vi "PXI Pnuematic Control.vi"(1 "Enable Relays":bool, 2 "Reset IO":bool, 3 "error in (no error)":errorcluster {"code" format="%.0x"}, 4 "Enum":T2(ring), 5 "topology name":T1="2566/16-SPDT", 6 "resource name":refnum<k15>="PXI1Slot6") -> (0 "error out":errorcluster)   [LabVIEW 2014]
uses:
  <instrlib>/niSwitch/niswitch.llb/niSwitch Relay Action.ctl
  <instrlib>/niSwitch/niswitch.llb/niSwitch Topologies.ctl
panel:
  out "instrument handle out":refnum<k15>
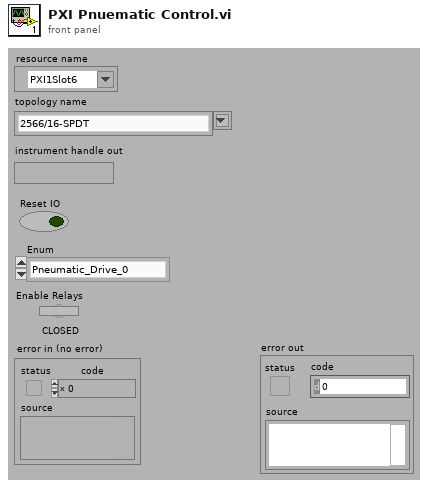
[diagram p1: front panel]
types:
  T1 = typedef "niSwitch Topologies.ctl" = string
  T2 = enum16{"Pneumatic_Drive_0", "Pneumatic_Drive_1", "Pneumatic_Drive_2", "Pneumatic_Drive_3", "Pneumatic_Drive_4", "Pneumatic_Drive_5", "Pneumatic_Drive_6", "Pneumatic_Drive_7", "Pneumatic_Drive_8", "Pneumatic_Drive_9", "Pneumatic_Drive_10", "Pneumatic_Drive_11", "Pneumatic_Drive_12", "Pneumatic_Drive_13", "Pneumatic_Drive_14", "Pneumatic_Drive_15", "Init Pneumatic Relays", "DeInit Pneumatic Relays"}
  T3 = typedef "niSwitch Relay Action.ctl" = i32
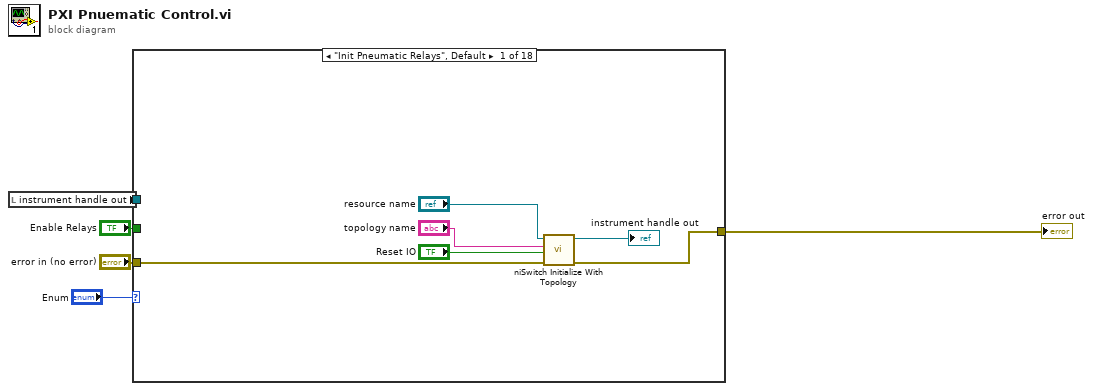
[diagram p0: block diagram]
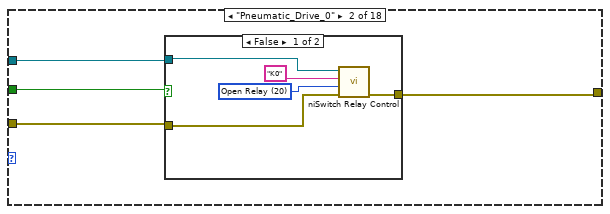
[diagram p2: hidden frame]
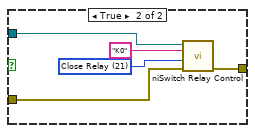
[diagram p3: hidden frame]
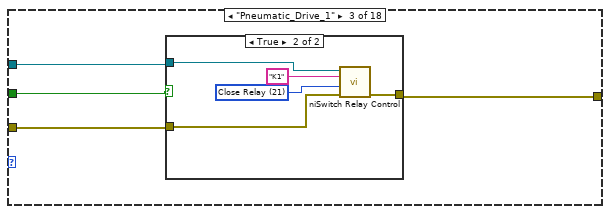
[diagram p4: hidden frame]
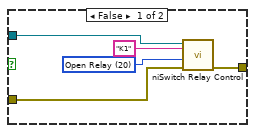
[diagram p5: hidden frame]
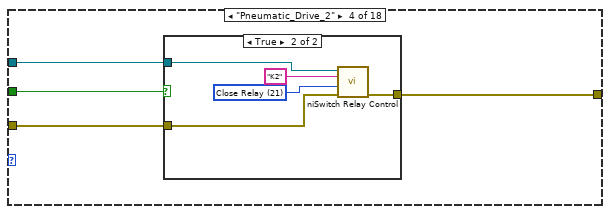
[diagram p6: hidden frame]
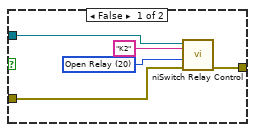
[diagram p7: hidden frame]
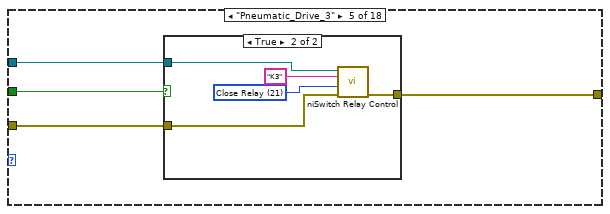
[diagram p8: hidden frame]
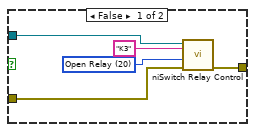
[diagram p9: hidden frame]
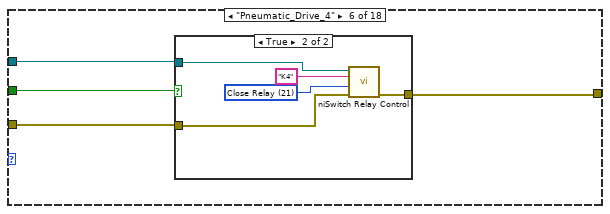
[diagram p10: hidden frame]
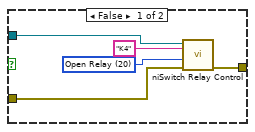
[diagram p11: hidden frame]
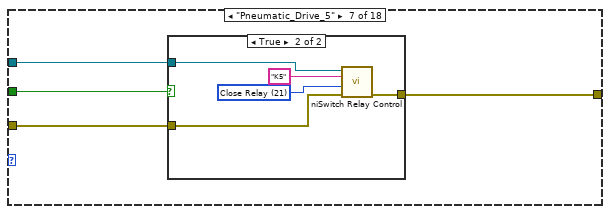
[diagram p12: hidden frame]
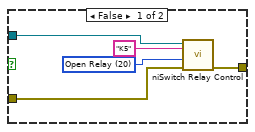
[diagram p13: hidden frame]
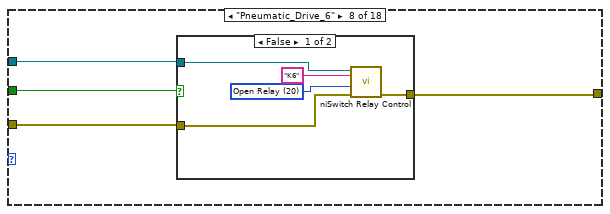
[diagram p14: hidden frame]
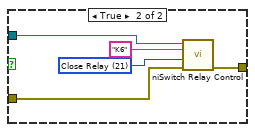
[diagram p15: hidden frame]
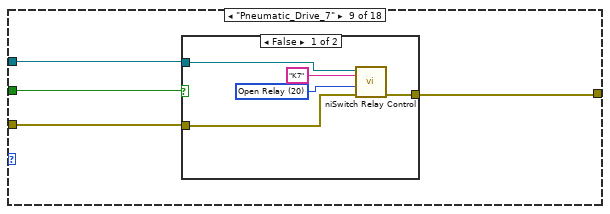
[diagram p16: hidden frame]
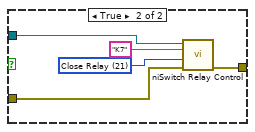
[diagram p17: hidden frame]
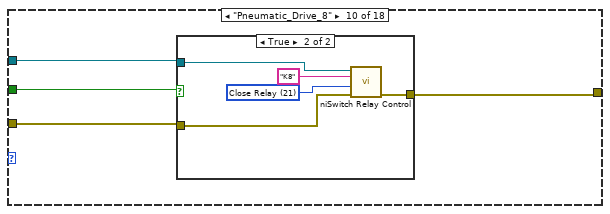
[diagram p18: hidden frame]
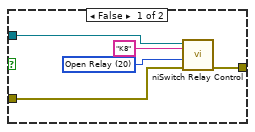
[diagram p19: hidden frame]
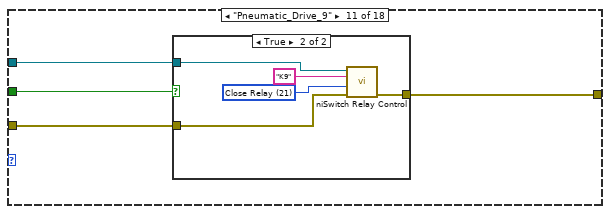
[diagram p20: hidden frame]
diagram:
  n1 = local read "instrument handle out"() -> (w4:refnum<k15>)
  n2 = case shown="\"Init Pneumatic Relays\", Default" "Enum" {
    tunnel: w4 -> [_ w15 w29 w43 w57 w71 w85 w99 w113 w127 w141 w155 w169 w183 w197 w211 w225 w238]
    tunnel: [w11 w12 w26 w40 w54 w68 w82 w96 w110 w124 w138 w152 w166 w180 w194 w208 w222 w236] -> w3
    tunnel: "Enable Relays" -> [_ w14 w27 w42 w56 w70 w84 w98 w112 w126 w140 w154 w168 w182 w196 w210 w224 _]
    tunnel: "error in (no error)" -> [w10 w13 w28 w41 w55 w69 w83 w97 w111 w125 w139 w153 w167 w181 w195 w209 w223 w237]
    frame "Init Pneumatic Relays", Default {
      n3 = call <instrlib>:"niSwitch Initialize With Topology.vi"("error in (no error)"=w10, "reset device (boolean value)"="Reset IO", "topology name"="topology name", "resource name"="resource name") -> ("error out"=w11:errorcluster, "instrument handle out"=→"instrument handle out":refnum<k15>)  [unwired: 6 in]
    }
    frame "Pneumatic_Drive_0" {
      n4 = case shown="False" w14 {
        tunnel: w15 -> [w18 w22]
        tunnel: [w19 w23] -> w12
        tunnel: w13 -> [w17 w21]
        frame False {
          w20 = T3 20 items=["Open Relay"=20, "Close Relay"=21] ("relay action (Close Relay)")
          n5 = call <instrlib>:"niSwitch Relay Control.vi"("error in (no error)"=w17, "relay action (Close Relay)"=w20, "relay name"="K0", "instrument handle"=w18) -> ("error out"=w19:errorcluster)  [unwired: 6 in, 1 out]
        }
        frame True {
          w25 = T3 21 items=["Open Relay"=20, "Close Relay"=21] ("relay action (Close Relay)")
          n6 = call <instrlib>:"niSwitch Relay Control.vi"("error in (no error)"=w21, "relay action (Close Relay)"=w25, "relay name"="K0", "instrument handle"=w22) -> ("error out"=w23:errorcluster)  [unwired: 6 in, 1 out]
        }
      }
    }
    frame "Pneumatic_Drive_1" {
      n7 = case shown="True" w27 {
        tunnel: w29 -> [w31 w36]
        tunnel: [w32 w37] -> w26
        tunnel: w28 -> [w30 w35]
        frame False {
          w34 = T3 20 items=["Open Relay"=20, "Close Relay"=21] ("relay action (Close Relay)")
          n8 = call <instrlib>:"niSwitch Relay Control.vi"("error in (no error)"=w30, "relay action (Close Relay)"=w34, "relay name"="K1", "instrument handle"=w31) -> ("error out"=w32:errorcluster)  [unwired: 6 in, 1 out]
        }
        frame True {
          w39 = T3 21 items=["Open Relay"=20, "Close Relay"=21] ("relay action (Close Relay)")
          n9 = call <instrlib>:"niSwitch Relay Control.vi"("error in (no error)"=w35, "relay action (Close Relay)"=w39, "relay name"="K1", "instrument handle"=w36) -> ("error out"=w37:errorcluster)  [unwired: 6 in, 1 out]
        }
      }
    }
    frame "Pneumatic_Drive_2" {
      n10 = case shown="True" w42 {
        tunnel: w43 -> [w45 w50]
        tunnel: [w46 w51] -> w40
        tunnel: w41 -> [w44 w49]
        frame False {
          w48 = T3 20 items=["Open Relay"=20, "Close Relay"=21] ("relay action (Close Relay)")
          n11 = call <instrlib>:"niSwitch Relay Control.vi"("error in (no error)"=w44, "relay action (Close Relay)"=w48, "relay name"="K2", "instrument handle"=w45) -> ("error out"=w46:errorcluster)  [unwired: 6 in, 1 out]
        }
        frame True {
          w53 = T3 21 items=["Open Relay"=20, "Close Relay"=21] ("relay action (Close Relay)")
          n12 = call <instrlib>:"niSwitch Relay Control.vi"("error in (no error)"=w49, "relay action (Close Relay)"=w53, "relay name"="K2", "instrument handle"=w50) -> ("error out"=w51:errorcluster)  [unwired: 6 in, 1 out]
        }
      }
    }
    frame "Pneumatic_Drive_3" {
      n13 = case shown="True" w56 {
        tunnel: w57 -> [w59 w64]
        tunnel: [w60 w65] -> w54
        tunnel: w55 -> [w58 w63]
        frame False {
          w62 = T3 20 items=["Open Relay"=20, "Close Relay"=21] ("relay action (Close Relay)")
          n14 = call <instrlib>:"niSwitch Relay Control.vi"("error in (no error)"=w58, "relay action (Close Relay)"=w62, "relay name"="K3", "instrument handle"=w59) -> ("error out"=w60:errorcluster)  [unwired: 6 in, 1 out]
        }
        frame True {
          w67 = T3 21 items=["Open Relay"=20, "Close Relay"=21] ("relay action (Close Relay)")
          n15 = call <instrlib>:"niSwitch Relay Control.vi"("error in (no error)"=w63, "relay action (Close Relay)"=w67, "relay name"="K3", "instrument handle"=w64) -> ("error out"=w65:errorcluster)  [unwired: 6 in, 1 out]
        }
      }
    }
    frame "Pneumatic_Drive_4" {
      n16 = case shown="True" w70 {
        tunnel: w71 -> [w73 w78]
        tunnel: [w74 w79] -> w68
        tunnel: w69 -> [w72 w77]
        frame False {
          w76 = T3 20 items=["Open Relay"=20, "Close Relay"=21] ("relay action (Close Relay)")
          n17 = call <instrlib>:"niSwitch Relay Control.vi"("error in (no error)"=w72, "relay action (Close Relay)"=w76, "relay name"="K4", "instrument handle"=w73) -> ("error out"=w74:errorcluster)  [unwired: 6 in, 1 out]
        }
        frame True {
          w81 = T3 21 items=["Open Relay"=20, "Close Relay"=21] ("relay action (Close Relay)")
          n18 = call <instrlib>:"niSwitch Relay Control.vi"("error in (no error)"=w77, "relay action (Close Relay)"=w81, "relay name"="K4", "instrument handle"=w78) -> ("error out"=w79:errorcluster)  [unwired: 6 in, 1 out]
        }
      }
    }
    frame "Pneumatic_Drive_5" {
      n19 = case shown="True" w84 {
        tunnel: w85 -> [w87 w92]
        tunnel: [w88 w93] -> w82
        tunnel: w83 -> [w86 w91]
        frame False {
          w90 = T3 20 items=["Open Relay"=20, "Close Relay"=21] ("relay action (Close Relay)")
          n20 = call <instrlib>:"niSwitch Relay Control.vi"("error in (no error)"=w86, "relay action (Close Relay)"=w90, "relay name"="K5", "instrument handle"=w87) -> ("error out"=w88:errorcluster)  [unwired: 6 in, 1 out]
        }
        frame True {
          w95 = T3 21 items=["Open Relay"=20, "Close Relay"=21] ("relay action (Close Relay)")
          n21 = call <instrlib>:"niSwitch Relay Control.vi"("error in (no error)"=w91, "relay action (Close Relay)"=w95, "relay name"="K5", "instrument handle"=w92) -> ("error out"=w93:errorcluster)  [unwired: 6 in, 1 out]
        }
      }
    }
    frame "Pneumatic_Drive_6" {
      n22 = case shown="False" w98 {
        tunnel: w99 -> [w101 w106]
        tunnel: [w102 w107] -> w96
        tunnel: w97 -> [w100 w105]
        frame False {
          w104 = T3 20 items=["Open Relay"=20, "Close Relay"=21] ("relay action (Close Relay)")
          n23 = call <instrlib>:"niSwitch Relay Control.vi"("error in (no error)"=w100, "relay action (Close Relay)"=w104, "relay name"="K6", "instrument handle"=w101) -> ("error out"=w102:errorcluster)  [unwired: 6 in, 1 out]
        }
        frame True {
          w109 = T3 21 items=["Open Relay"=20, "Close Relay"=21] ("relay action (Close Relay)")
          n24 = call <instrlib>:"niSwitch Relay Control.vi"("error in (no error)"=w105, "relay action (Close Relay)"=w109, "relay name"="K6", "instrument handle"=w106) -> ("error out"=w107:errorcluster)  [unwired: 6 in, 1 out]
        }
      }
    }
    frame "Pneumatic_Drive_7" {
      n25 = case shown="False" w112 {
        tunnel: w113 -> [w115 w120]
        tunnel: [w116 w121] -> w110
        tunnel: w111 -> [w114 w119]
        frame False {
          w118 = T3 20 items=["Open Relay"=20, "Close Relay"=21] ("relay action (Close Relay)")
          n26 = call <instrlib>:"niSwitch Relay Control.vi"("error in (no error)"=w114, "relay action (Close Relay)"=w118, "relay name"="K7", "instrument handle"=w115) -> ("error out"=w116:errorcluster)  [unwired: 6 in, 1 out]
        }
        frame True {
          w123 = T3 21 items=["Open Relay"=20, "Close Relay"=21] ("relay action (Close Relay)")
          n27 = call <instrlib>:"niSwitch Relay Control.vi"("error in (no error)"=w119, "relay action (Close Relay)"=w123, "relay name"="K7", "instrument handle"=w120) -> ("error out"=w121:errorcluster)  [unwired: 6 in, 1 out]
        }
      }
    }
    frame "Pneumatic_Drive_8" {
      n28 = case shown="True" w126 {
        tunnel: w127 -> [w129 w134]
        tunnel: [w130 w135] -> w124
        tunnel: w125 -> [w128 w133]
        frame False {
          w132 = T3 20 items=["Open Relay"=20, "Close Relay"=21] ("relay action (Close Relay)")
          n29 = call <instrlib>:"niSwitch Relay Control.vi"("error in (no error)"=w128, "relay action (Close Relay)"=w132, "relay name"="K8", "instrument handle"=w129) -> ("error out"=w130:errorcluster)  [unwired: 6 in, 1 out]
        }
        frame True {
          w137 = T3 21 items=["Open Relay"=20, "Close Relay"=21] ("relay action (Close Relay)")
          n30 = call <instrlib>:"niSwitch Relay Control.vi"("error in (no error)"=w133, "relay action (Close Relay)"=w137, "relay name"="K8", "instrument handle"=w134) -> ("error out"=w135:errorcluster)  [unwired: 6 in, 1 out]
        }
      }
    }
    frame "Pneumatic_Drive_9" {
      n31 = case shown="True" w140 {
        tunnel: w141 -> [w143 w148]
        tunnel: [w144 w149] -> w138
        tunnel: w139 -> [w142 w147]
        frame False {
          w146 = T3 20 items=["Open Relay"=20, "Close Relay"=21] ("relay action (Close Relay)")
          n32 = call <instrlib>:"niSwitch Relay Control.vi"("error in (no error)"=w142, "relay action (Close Relay)"=w146, "relay name"="K9", "instrument handle"=w143) -> ("error out"=w144:errorcluster)  [unwired: 6 in, 1 out]
        }
        frame True {
          w151 = T3 21 items=["Open Relay"=20, "Close Relay"=21] ("relay action (Close Relay)")
          n33 = call <instrlib>:"niSwitch Relay Control.vi"("error in (no error)"=w147, "relay action (Close Relay)"=w151, "relay name"="K9", "instrument handle"=w148) -> ("error out"=w149:errorcluster)  [unwired: 6 in, 1 out]
        }
      }
    }
    frame "Pneumatic_Drive_10" {
      n34 = case shown="True" w154 {
        tunnel: w155 -> [w157 w162]
        tunnel: [w158 w163] -> w152
        tunnel: w153 -> [w156 w161]
        frame False {
          w160 = T3 20 items=["Open Relay"=20, "Close Relay"=21] ("relay action (Close Relay)")
          n35 = call <instrlib>:"niSwitch Relay Control.vi"("error in (no error)"=w156, "relay action (Close Relay)"=w160, "relay name"="K10", "instrument handle"=w157) -> ("error out"=w158:errorcluster)  [unwired: 6 in, 1 out]
        }
        frame True {
          w165 = T3 21 items=["Open Relay"=20, "Close Relay"=21] ("relay action (Close Relay)")
          n36 = call <instrlib>:"niSwitch Relay Control.vi"("error in (no error)"=w161, "relay action (Close Relay)"=w165, "relay name"="K10", "instrument handle"=w162) -> ("error out"=w163:errorcluster)  [unwired: 6 in, 1 out]
        }
      }
    }
    frame "Pneumatic_Drive_11" {
      n37 = case shown="True" w168 {
        tunnel: w169 -> [w171 w176]
        tunnel: [w172 w177] -> w166
        tunnel: w167 -> [w170 w175]
        frame False {
          w174 = T3 20 items=["Open Relay"=20, "Close Relay"=21] ("relay action (Close Relay)")
          n38 = call <instrlib>:"niSwitch Relay Control.vi"("error in (no error)"=w170, "relay action (Close Relay)"=w174, "relay name"="K11", "instrument handle"=w171) -> ("error out"=w172:errorcluster)  [unwired: 6 in, 1 out]
        }
        frame True {
          w179 = T3 21 items=["Open Relay"=20, "Close Relay"=21] ("relay action (Close Relay)")
          n39 = call <instrlib>:"niSwitch Relay Control.vi"("error in (no error)"=w175, "relay action (Close Relay)"=w179, "relay name"="K11", "instrument handle"=w176) -> ("error out"=w177:errorcluster)  [unwired: 6 in, 1 out]
        }
      }
    }
    frame "Pneumatic_Drive_12" {
      n40 = case shown="True" w182 {
        tunnel: w183 -> [w185 w190]
        tunnel: [w186 w191] -> w180
        tunnel: w181 -> [w184 w189]
        frame False {
          w188 = T3 20 items=["Open Relay"=20, "Close Relay"=21] ("relay action (Close Relay)")
          n41 = call <instrlib>:"niSwitch Relay Control.vi"("error in (no error)"=w184, "relay action (Close Relay)"=w188, "relay name"="K12", "instrument handle"=w185) -> ("error out"=w186:errorcluster)  [unwired: 6 in, 1 out]
        }
        frame True {
          w193 = T3 21 items=["Open Relay"=20, "Close Relay"=21] ("relay action (Close Relay)")
          n42 = call <instrlib>:"niSwitch Relay Control.vi"("error in (no error)"=w189, "relay action (Close Relay)"=w193, "relay name"="K12", "instrument handle"=w190) -> ("error out"=w191:errorcluster)  [unwired: 6 in, 1 out]
        }
      }
    }
    frame "Pneumatic_Drive_13" {
      n43 = case shown="False" w196 {
        tunnel: w197 -> [w199 w204]
        tunnel: [w200 w205] -> w194
        tunnel: w195 -> [w198 w203]
        frame False {
          w202 = T3 20 items=["Open Relay"=20, "Close Relay"=21] ("relay action (Close Relay)")
          n44 = call <instrlib>:"niSwitch Relay Control.vi"("error in (no error)"=w198, "relay action (Close Relay)"=w202, "relay name"="K13", "instrument handle"=w199) -> ("error out"=w200:errorcluster)  [unwired: 6 in, 1 out]
        }
        frame True {
          w207 = T3 21 items=["Open Relay"=20, "Close Relay"=21] ("relay action (Close Relay)")
          n45 = call <instrlib>:"niSwitch Relay Control.vi"("error in (no error)"=w203, "relay action (Close Relay)"=w207, "relay name"="K13", "instrument handle"=w204) -> ("error out"=w205:errorcluster)  [unwired: 6 in, 1 out]
        }
      }
    }
    frame "Pneumatic_Drive_14" {
      n46 = case shown="True" w210 {
        tunnel: w211 -> [w213 w218]
        tunnel: [w214 w219] -> w208
        tunnel: w209 -> [w212 w217]
        frame False {
          w216 = T3 20 items=["Open Relay"=20, "Close Relay"=21] ("relay action (Close Relay)")
          n47 = call <instrlib>:"niSwitch Relay Control.vi"("error in (no error)"=w212, "relay action (Close Relay)"=w216, "relay name"="K14", "instrument handle"=w213) -> ("error out"=w214:errorcluster)  [unwired: 6 in, 1 out]
        }
        frame True {
          w221 = T3 21 items=["Open Relay"=20, "Close Relay"=21] ("relay action (Close Relay)")
          n48 = call <instrlib>:"niSwitch Relay Control.vi"("error in (no error)"=w217, "relay action (Close Relay)"=w221, "relay name"="K14", "instrument handle"=w218) -> ("error out"=w219:errorcluster)  [unwired: 6 in, 1 out]
        }
      }
    }
    frame "Pneumatic_Drive_15" {
      n49 = case shown="False" w224 {
        tunnel: w225 -> [w227 w232]
        tunnel: [w228 w233] -> w222
        tunnel: w223 -> [w226 w231]
        frame False {
          w230 = T3 20 items=["Open Relay"=20, "Close Relay"=21] ("relay action (Close Relay)")
          n50 = call <instrlib>:"niSwitch Relay Control.vi"("error in (no error)"=w226, "relay action (Close Relay)"=w230, "relay name"="K15", "instrument handle"=w227) -> ("error out"=w228:errorcluster)  [unwired: 6 in, 1 out]
        }
        frame True {
          w235 = T3 21 items=["Open Relay"=20, "Close Relay"=21] ("relay action (Close Relay)")
          n51 = call <instrlib>:"niSwitch Relay Control.vi"("error in (no error)"=w231, "relay action (Close Relay)"=w235, "relay name"="K15", "instrument handle"=w232) -> ("error out"=w233:errorcluster)  [unwired: 6 in, 1 out]
        }
      }
    }
    frame "DeInit Pneumatic Relays" {
      n52 = call <instrlib>:"niSwitch Close.vi"("error in (no error)"=w237, "instrument handle"=w238) -> ("error out"=w236:errorcluster)  [unwired: 9 in]
    }
  }
  "error out" <- w3
